vi "Transformation Matrix to Transform Components.vi"(0 "4x4 Transformation Matrix":T2) -> (1 "tvec":T1, 2 "Rotation Matrix":T2)   [LabVIEW 2020, in "ar.lvlib"]
doc: "Convert a 4x4 Transformation Matrix to a 3D Pose."
uses:
  ar.lvlib
  tvec.ctl
  <vilib>/Analysis/Matrix/Datatypes/RealMatrix.ctl
  <vilib>/Analysis/Matrix/NI_Matrix.lvlib
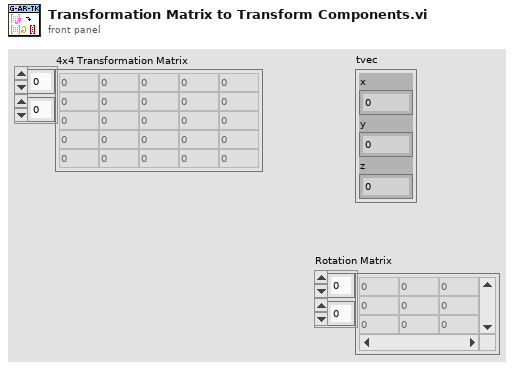
[diagram p1: front panel]
types:
  T1 = typedef "ar.lvlib/tvec.ctl" = cluster{"x":dbl, "y":dbl, "z":dbl}
  T2 = typedef "NI_Matrix.lvlib/RealMatrix.ctl" = dbl[][]
  T3 = cluster{"4x4 Transformation Matrix[0]":dbl, "4x4 Transformation Matrix[1]":dbl, "4x4 Transformation Matrix[2]":dbl}
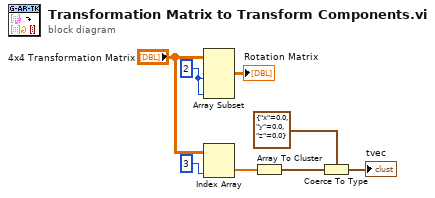
[diagram p0: block diagram]
diagram:
  w8 = 2 ("row N")
  n1 = Array Subset(array="4x4 Transformation Matrix", length (row)=w8, length (col)=w8) -> (→"Rotation Matrix":T2)  [unwired: 2 in]
  n2 = Index Array(array="4x4 Transformation Matrix", index (col)=3 ("disabled index (col)")) -> (element=w5:dbl[])  [unwired: 1 in]
  n3 = Array To Cluster(array=w5) -> (cluster=w4:T3)
  n4 = Coerce To Type(0:w4, 1:T1 {"x"=0.0, "y"=0.0, "z"=0.0} ("tvec")) -> (2:→"tvec":T1)
